vi "Switch Open Refs.vi"(8 "error in":errorcluster, 11 "CSV File":path=path "C:/Users/chericks/Desktop/P2_Module/P2_Module/Test Code/Test_Sense_Routes.csv") -> (0 "error out":errorcluster, 3 "Switch Refs":refnum<k15>[](array[refnum]))   [LabVIEW 2019]
uses:
  <instrlib>/niSwitch/niSwitch.llb/niSwitch Topologies.ctl
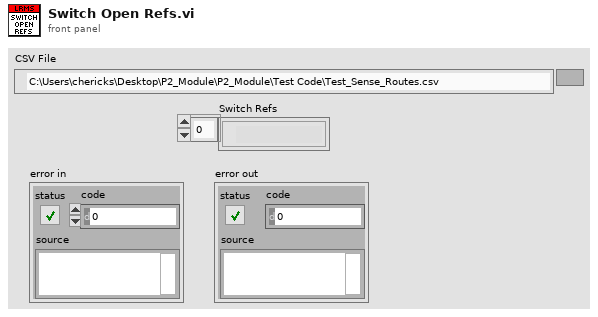
[diagram p1: front panel]
types:
  T1 = typedef "niSwitch Topologies.ctl" = string
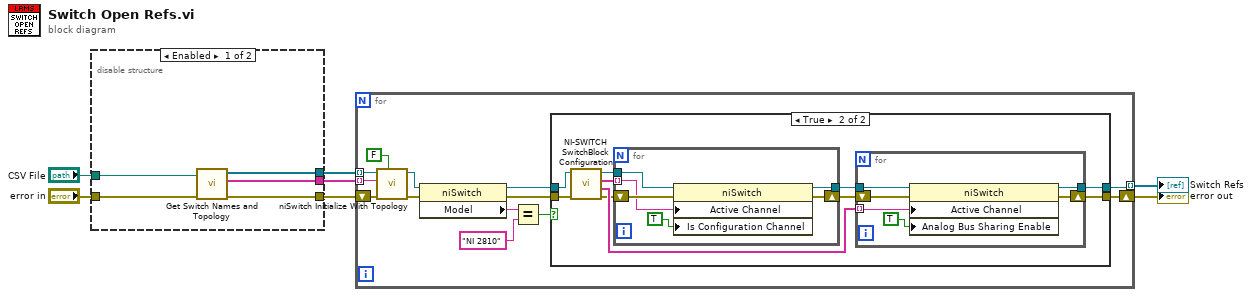
[diagram p0: block diagram]
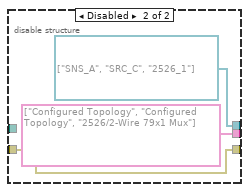
[diagram p2: hidden frame]
diagram:
  n1 = disable-structure shown="Enabled" {
    disable-tunnel: [w12 refnum<k15>[] ["SNS_A", "SRC_C", "2526_1"]] -> w5
    disable-tunnel: [w11 T1[] ["Configured Topology", "Configured Topology", "2526/2-Wire 79x1 Mux"]] -> w4
    disable-tunnel: [w10 w13] -> w3
    disable-tunnel: "error in" -> [w9 w13]
    disable-tunnel: "CSV File" -> [w8 _]
    frame Enabled {
      n2 = call "Get Switch Names and Topology.vi"("error in (no error)"=w9, "CSV File"=w8) -> ("error out"=w10:errorcluster, "Switch Topologies"=w11:T1[], "Switch Resource Names"=w12:refnum<k15>[])  [unwired: 7 in]
    }
    frame Disabled {
    }
  }
  n3 = for {
    tunnel: w5 -> [w28] mode=indexing
    shift-right: [w18] -> w7
    shift-left: w3 -> [w26]
    tunnel: [w17] -> w6 mode=indexing
    tunnel: w4 -> [w16] mode=indexing
    n4 = call <instrlib>:"niSwitch Initialize With Topology.vi"("simulate (boolean value)"=FALSE, "error in (no error)"=w26, "topology name"=w16, "resource name"=w28) -> ("error out"=w24:errorcluster, "instrument handle out"=w25:refnum<k15>)  [unwired: 6 in]
    n5 = property class="niSwitch"(reference=w25, error in=w24) -> (reference out=w22:refnum<k15>, error out=w23:errorcluster, "Model"=w21:string)
    n6 = Equal?(x=w21, y="NI 2810") -> (x = y?=w19:bool)
    n7 = case shown="True" w19 {
      tunnel: [w30 w37] -> w17
      tunnel: [w29 w36] -> w18
      tunnel: w23 -> [w29 w34]
      tunnel: w22 -> [w30 w33]
      frame False {
      }
      frame True {
        n8 = call "NI-SWITCH SwitchBlock Configuration.vi"("error in (no error)"=w34, "Reference In"=w33) -> ("error out"=w31:errorcluster, "Analog Bus Array"=w32:string[], "Row Array"=w39:string[], "Reference out"=w35:refnum<k15>)  [unwired: 6 in]
        n9 = for {
          tunnel: w39 -> [w49] mode=indexing
          shift-right: [w51] -> w38
          shift-left: w31 -> [w50]
          tunnel: w35 -> [w48]
          tunnel: [w47] -> w40
          n10 = property class="niSwitch"(reference=w48, error in=w50, "Active Channel"=w49, "Is Configuration Channel"=TRUE ("Channel Configuration:Is Configuration Channel")) -> (reference out=w47:refnum<k15>, error out=w51:errorcluster)
        }
        n11 = for {
          shift-right: [w43] -> w36
          shift-left: w38 -> [w44]
          tunnel: w40 -> [w45]
          tunnel: [w42] -> w37
          tunnel: w32 -> [w41] mode=indexing
          n12 = property class="niSwitch"(reference=w45, error in=w44, "Active Channel"=w41, "Analog Bus Sharing Enable"=TRUE ("Channel Configuration:Is Configuration Channel")) -> (reference out=w42:refnum<k15>, error out=w43:errorcluster)
        }
      }
    }
  }
  "Switch Refs" <- w6
  "error out" <- w7
